vi "pose - XML.vi"(8 "tag":string, 10 "T":T1=[[0.016284994521607307, 0.9998576764567041, 0.0044074691186384496, -12.095922523672678], [0.9998670931969393, -0.01628143110047913, -0.0008431744914288715, -1019.3924117975101], [-0.0007712945830650122, 0.004420614427981981, -0.999989931585686, 240.25900755427352], [0.0, 0.0, 0.0, 1.0]] format="%.3f", 11 "Object":string) -> (3 "String":string)   [LabVIEW 2013]
uses:
  <vilib>/Analysis/Matrix/Datatypes/RealMatrix.ctl
  <vilib>/Analysis/Matrix/NI_Matrix.lvlib
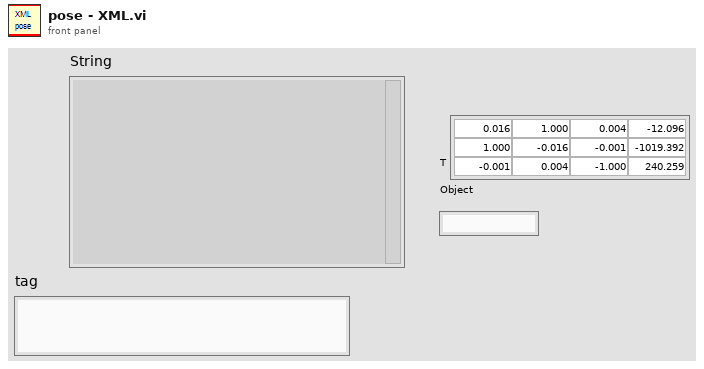
[diagram p1: front panel]
types:
  T1 = typedef "NI_Matrix.lvlib/RealMatrix.ctl" = dbl[][]
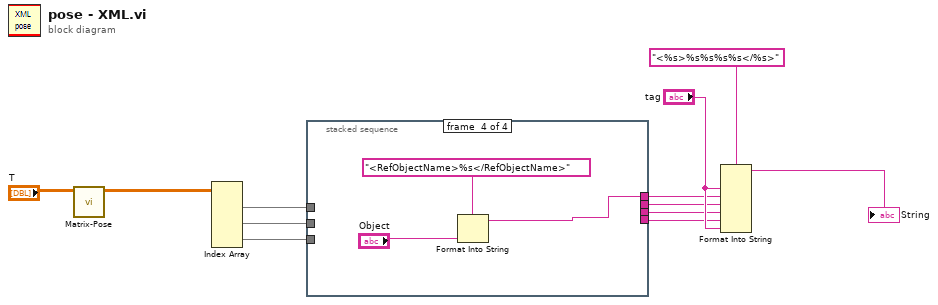
[diagram p0: block diagram]
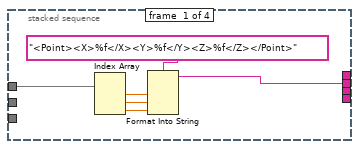
[diagram p2: hidden frame]
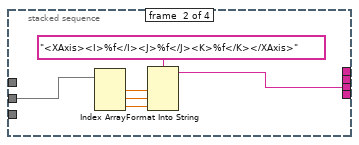
[diagram p3: hidden frame]
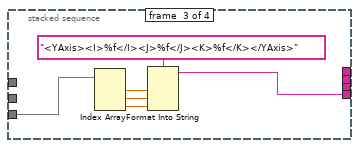
[diagram p4: hidden frame]
diagram:
  n1 = call "Matrix-Pose.vi"("T"="T") -> ("pose"=w11:dbl[][])  [unwired: 9 in, 1 out]
  n2 = Index Array(array=w11) -> (element #1=w10:dbl[], element #2=w9:dbl[], element #3=w8:dbl[])  [unwired: 6 in]
  n3 = stacked-sequence {
    tunnel: w10 -> [w17 _ _ _]
    tunnel: w9 -> [_ w21 _ _]
    tunnel: w8 -> [_ _ w26 _]
    tunnel: [w13 _ _ _] -> w3
    tunnel: [_ w19 _ _] -> w2
    tunnel: [_ _ w25 _] -> w1
    tunnel: [_ _ _ w31] -> w4
    frame #0 {
      n4 = Index Array(array=w17) -> (element #1=w16:dbl, element #2=w15:dbl, element #3=w14:dbl)  [unwired: 3 in]
      n5 = Format Into String(format string="<Point><X>%f</X><Y>%f</Y><Z>%f</Z></Point>", w16, w15, w14) -> (resulting string=w13:string)  [unwired: 2 in, 1 out]
    }
    frame #1 {
      n6 = Index Array(array=w21) -> (element #1=w24:dbl, element #2=w23:dbl, element #3=w22:dbl)  [unwired: 3 in]
      n7 = Format Into String(format string="<XAxis><I>%f</I><J>%f</J><K>%f</K></XAxis>", w24, w23, w22) -> (resulting string=w19:string)  [unwired: 2 in, 1 out]
    }
    frame #2 {
      n8 = Index Array(array=w26) -> (element #1=w30:dbl, element #2=w29:dbl, element #3=w28:dbl)  [unwired: 3 in]
      n9 = Format Into String(format string="<YAxis><I>%f</I><J>%f</J><K>%f</K></YAxis>", w30, w29, w28) -> (resulting string=w25:string)  [unwired: 2 in, 1 out]
    }
    frame #3 {
      n10 = Format Into String(format string="<RefObjectName>%s</RefObjectName>" ("tag"), "Object") -> (resulting string=w31:string)  [unwired: 2 in, 1 out]
    }
  }
  n11 = Format Into String(format string="<%s>%s%s%s%s</%s>", "tag", w4, w3, w2, w1, "tag") -> (resulting string=→"String":string)  [unwired: 2 in, 1 out]
